vi "Write My Data to TDMS.vi"(4 "Data":T1(array[cluster]), 5 "Comment":string, 7 "Time Stamp":timestamp, 8 "error in":errorcluster, 10 "Dataset Path":string, 11 "file path":path) -> (0 "error out":errorcluster)   [LabVIEW 2014]
panel:
  in  "Good":bool
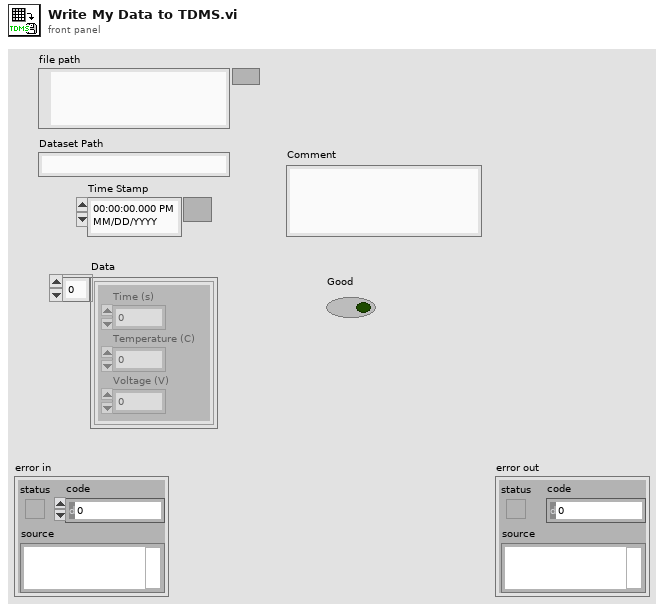
[diagram p1: front panel]
types:
  T1 = cluster{"Time (s)":dbl, "Temperature (C)":dbl, "Voltage (V)":dbl}[]
  T2 = enum16{"open", "open or create", "create or replace", "create", "open (read-only)"}
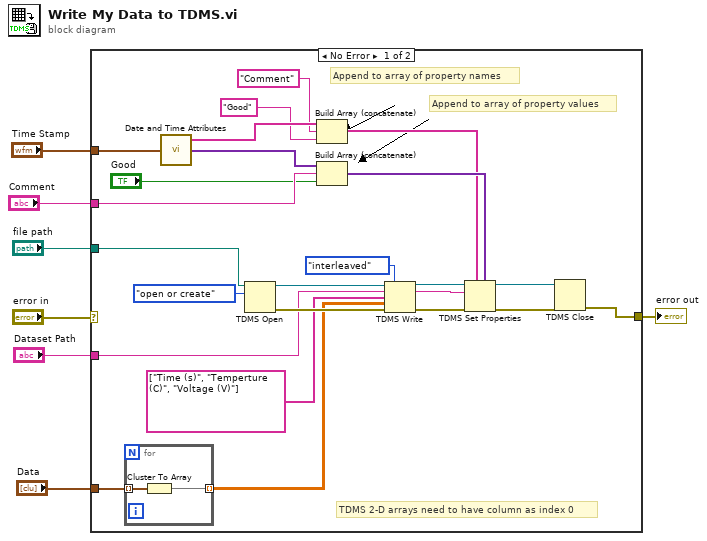
[diagram p0: block diagram]
diagram:
  n1 = case shown="No Error" "error in" {
    selector: "error in" -> [_ w34]
    tunnel: [w10 w34] -> w7
    tunnel: "file path" -> [w21 _]
    tunnel: "Time Stamp" -> [w31 _]
    tunnel: "Comment" -> [w27 _]
    tunnel: "Dataset Path" -> [w19 _]
    tunnel: "Data" -> [w24 _]
    frame No Error {
      # "TDMS 2-D arrays need to have column as index 0"
      # "Append to array of property values"
      # "Append to array of property names"
      n2 = for {
        tunnel: w24 -> [w33] mode=indexing
        tunnel: [w32] -> w8 mode=indexing
        n3 = Cluster To Array(cluster=w33) -> (array=w32:dbl[])
      }
      n4 = call <vilib>:"Date and Time Attributes.vi"("Timestamp (current)"=w31) -> ("Attribute Names"=w30:string[], "Attribute Values"=w28:variant[])  [unwired: 1 out]
      n5 = TDMS Open(10:T2."open or create" ("operation (0:open)"), 11:w21) -> (0:w22:errorcluster, 3:w23:refnum<k34>)  [unwired: 5 in]
      n6 = Build Array (concatenate)(w30, "Comment", "Good" ("element")) -> (w13:string[])
      n7 = Build Array (concatenate)(w28, w27, "Good") -> (w14:variant[])
      n8 = TDMS Write(0:w23, 1:enum16{"decimated", "interleaved"}."interleaved" ("data layout (0:decimated)"), 5:w19, 7:string[] ["Time (s)", "Temperture (C)", "Voltage (V)"], 9:w8, 11:w22) -> (4:w17:refnum<k34>, 6:w16:string, 15:w15:errorcluster)  [unwired: 1 out]
      n9 = TDMS Set Properties(5:w14, 7:w13, 8:w15, 10:w16, 11:w17) -> (0:w12:errorcluster, 3:w11:refnum<k34>)  [unwired: 1 in, 2 out]
      n10 = TDMS Close(8:w12, 11:w11) -> (0:w10:errorcluster)  [unwired: 1 out]
    }
    frame Error {
      # "Wire previous error through"
    }
  }
  "error out" <- w7
